vi "Set Tag.vi"(8 "error in (no error)":errorcluster, 9 "Variant":variant, 10 "tag (case insensitive)":string, 11 "uData in":refnum<class "uData.lvclass">) -> (0 "error out":errorcluster, 3 "uData out":refnum<class "uData.lvclass">, 4 "replaced?":bool)   [LabVIEW 2023, in "uLib.lvlib" / "uData.lvclass"]
doc: "Append a new tag or replace an existing tag."
uses:
  uData.lvclass
  uData.lvclass/uData.ctl
  Blank Key Reserved String.vi
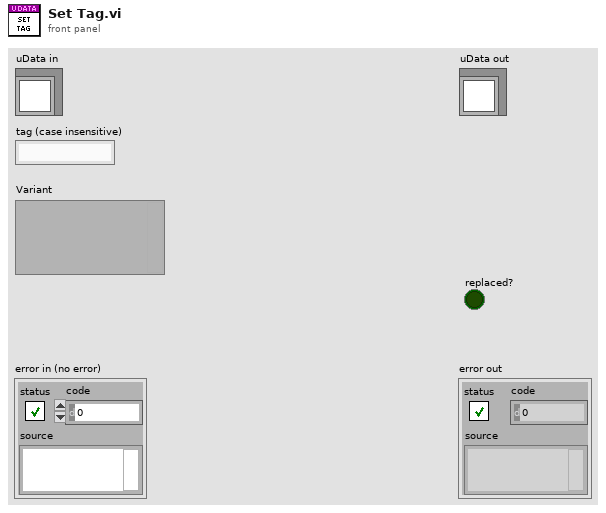
[diagram p1: front panel]
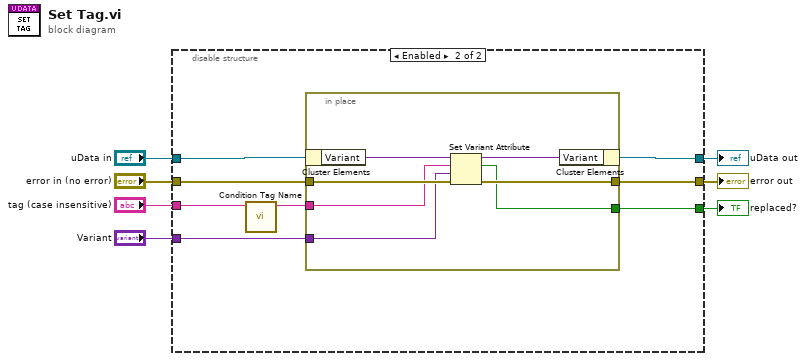
[diagram p0: block diagram]
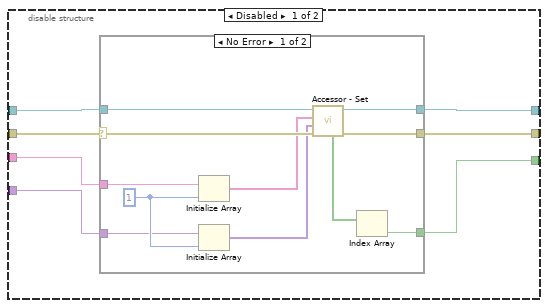
[diagram p2: hidden frame]
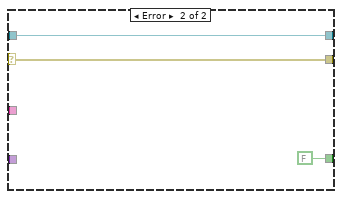
[diagram p3: hidden frame]
diagram:
  n1 = disable-structure shown="Enabled" {
    disable-tunnel: "uData in" -> [w14 w36]
    disable-tunnel: [w13 w35] -> w6
    disable-tunnel: [w12 w34] -> w5
    disable-tunnel: [w11 w32] -> w4
    disable-tunnel: "tag (case insensitive)" -> [w10 w31]
    disable-tunnel: "Variant" -> [w9 w29]
    disable-tunnel: "error in (no error)" -> [w8 w33]
    frame Disabled {
      n2 = case shown="No Error" w8 {
        selector: w8 -> [w24 w28]
        tunnel: w14 -> [w23 w27]
        tunnel: [w22 w27] -> w13
        tunnel: [w25 w28] -> w12
        tunnel: [w20 FALSE ("replaced")] -> w11
        tunnel: w10 -> [w18 _]
        tunnel: w9 -> [w15 _]
        frame No Error {
          w19 = 1 ("dimension size")
          n3 = Initialize Array(w18, w19) -> (w17:string[])
          n4 = Initialize Array(w15, w19) -> (w16:variant[])
          n5 = call "Accessor - Set.vi"("error in (no error)"=w24, "values"=w16, "keys"=w17, "uData in"=w23) -> ("error out"=w25:errorcluster, "uData out"=w22:refnum<class "uData.lvclass">, "replaced?"=w21:bool[])  [unwired: 5 in]
          n6 = Index Array(array=w21) -> (element=w20:bool)  [unwired: 1 in]
        }
        frame Error {
        }
      }
    }
    frame Enabled {
      n7 = call "Condition Tag Name.vi"("tag in"=w31) -> ("tag out"=w30:string)  [unwired: 10 in]
      n8 = in-place {
        in-place-border: [w41] -> w34
        in-place-border: w33 -> [w40]
        in-place-border: [w39] -> w32
        in-place-border: w30 -> [w37]
        in-place-border: w29 -> [w38]
        n9 = in-place-cluster #1(w36) -> ("Variant"=w43:variant)
        n10 = Set Variant Attribute(Variant=w43, name=w37, value=w38, error in=w40) -> (Variant out=w42:variant, replaced=w39:bool, error out=w41:errorcluster)
        n11 = in-place-cluster #1("Variant"=w42) -> (w35:refnum<class "uData.lvclass">)
      }
    }
  }
  "error out" <- w5
  "uData out" <- w6
  "replaced?" <- w4
